vi "Test Write in Loop.vi"() -> ()   [LabVIEW 2014, in "Arduino SoftwareSerial Wrapper.lvlib"]
uses:
  Arduino SoftwareSerial Wrapper.lvlib
panel:
  out "Error Out":errorcluster
  in  "Error In":errorcluster
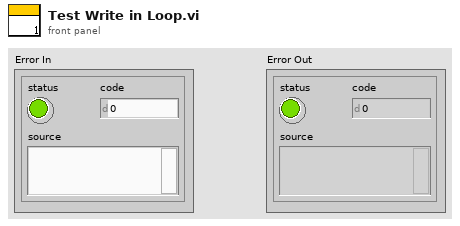
[diagram p1: front panel]
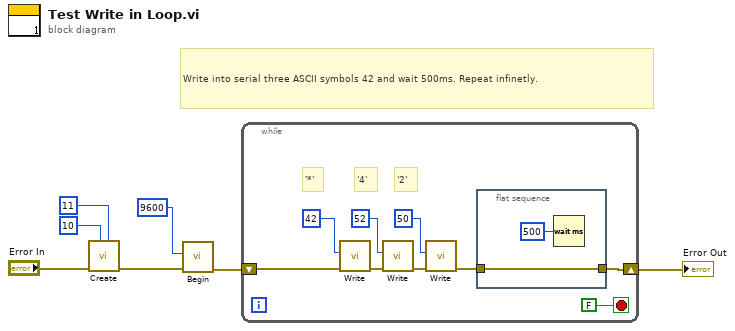
[diagram p0: block diagram]
diagram:
  # "Write into serial three ASCII symbols 42 and wait 500ms. Repeat infinetly."
  n1 = call "Create.vi"("arduino RX pin"=u8 11 ("RX pin"), "arduino TX pin"=u8 10 ("RX pin"), "Error In"="Error In") -> ("Error Out"=w3:errorcluster)  [unwired: 8 in]
  n2 = call "Begin.vi"("Error In"=w3, "Baudrate"=u16 9600) -> ("Error Out"=w2:errorcluster)  [unwired: 8 in]
  n3 = while {
    shift-right: [w11] -> w4
    shift-left: w2 -> [w8]
    stop <- FALSE stop-if-true
    # "'2'"
    # "'4'"
    # "'*'"
    n4 = call "Write.vi"("Error In"=w8, "Char to write"=u8 42) -> ("Error Out"=w13:errorcluster)  [unwired: 9 in]
    n5 = call "Write.vi"("Error In"=w13, "Char to write"=u8 52) -> ("Error Out"=w12:errorcluster)  [unwired: 9 in]
    n6 = call "Write.vi"("Error In"=w12, "Char to write"=u8 50) -> ("Error Out"=w10:errorcluster)  [unwired: 9 in]
    n7 = flat-sequence {
      tunnel: [w18] -> w11
      tunnel: w10 -> [w18]
      frame #0 {
        n8 = Wait (ms)(milliseconds to wait=u32 500) -> ()  [unwired: 1 out]
      }
    }
  }
  "Error Out" <- w4
